vi "Pickering 4 Wire PPMS DR Asynchronous.vi"(8 "error in (no error)":errorcluster, 10 "Channel Cluster":T1, 11 "Control Experiment in":refnum<class "Control Experiment.lvclass">) -> (0 "error out":errorcluster, 3 "Control Experiment out":refnum<class "Control Experiment.lvclass">)   [LabVIEW 2016, in "Control Experiment.lvclass"]
uses:
  Control Experiment.lvclass
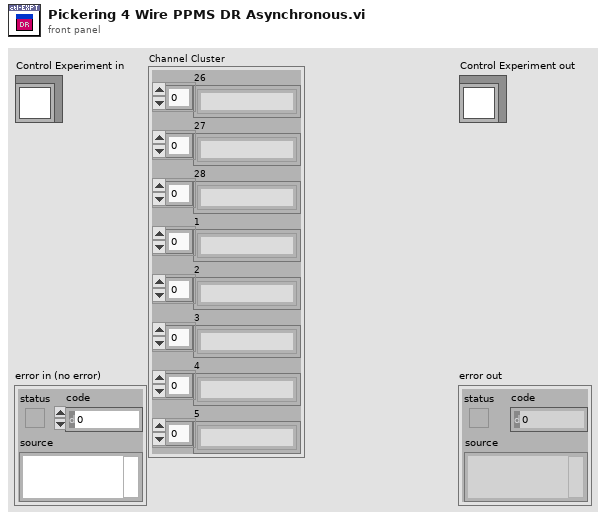
[diagram p1: front panel]
types:
  T1 = cluster{"26":string[], "27":string[], "28":string[], "1":string[], "2":string[], "3":string[], "4":string[], "5":string[]}
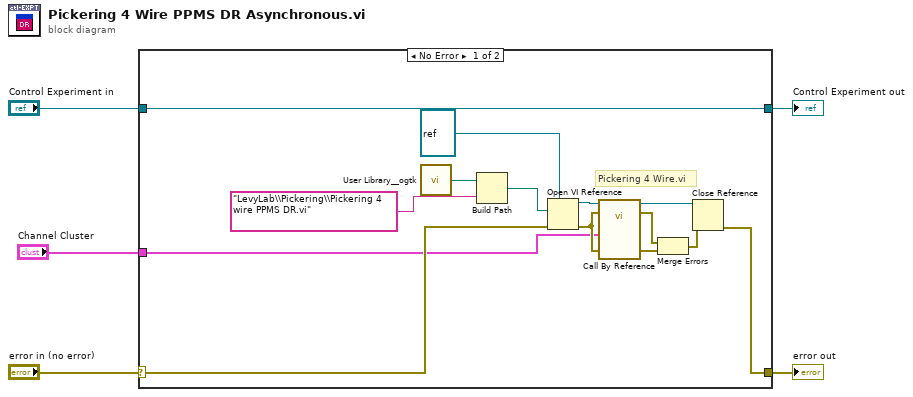
[diagram p0: block diagram]
diagram:
  n1 = case shown="No Error" "error in (no error)" {
    selector: "error in (no error)" -> [w10 w21]
    tunnel: [w9 w21] -> w4
    tunnel: [w19 w20] -> w2
    tunnel: "Control Experiment in" -> [w19 w20]
    tunnel: "Channel Cluster" -> [w6 _]
    frame No Error {
      # "Pickering 4 Wire.vi"
      n2 = call <userlib>:"User Library__ogtk.vi"() -> ("User Library (+ Relative)"=w13:path)  [unwired: 1 in]
      n3 = Build Path(base path=w13, name or relative path="LevyLab\\Pickering\\Pickering 4 wire PPMS DR.vi") -> (appended path=w11:path)
      n4 = Open VI Reference(type specifier VI Refnum (for type only)=refnum<vi> refnum, vi path=w11, error in (no error)=w10) -> (vi reference=w18:refnum<vi>, error out=w12:errorcluster)  [unwired: 3 in]
      n5 = call-by-ref "?"(reference=w18, error in=w12, 8:"error in (no error)"=w12, "Channel Cluster"=w6) -> (reference out=w17:refnum<vi>, error out=w16:errorcluster, 0:"error out"=w15:errorcluster)  [unwired: 9 in]
      n6 = Merge Errors(w16, w15) -> (w14:errorcluster)
      n7 = Close Reference(reference=w17, error in (no error)=w14) -> (error out=w9:errorcluster)
    }
    frame Error {
    }
  }
  "error out" <- w4
  "Control Experiment out" <- w2
